vi "Create Three Input  Data Table.vi"(8 "错误输入（无错误）":errorcluster, 9 "Result":bool[](array[boolean]), 10 "Data":bool[][](array[boolean]), 11 "Data Table Ref In":refnum<vi>) -> (0 "错误输出":errorcluster, 3 "Data Table Ref Out":refnum<vi>)   [LabVIEW 2012]
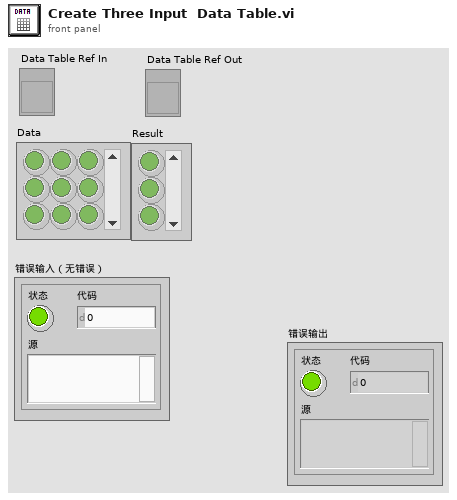
[diagram p1: front panel]
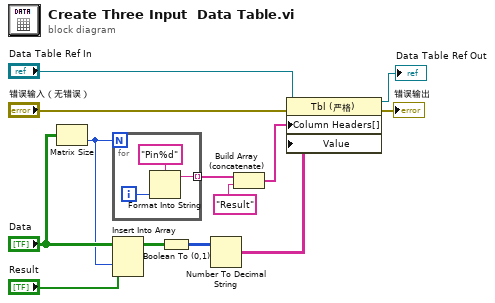
[diagram p0: block diagram]
diagram:
  n1 = Matrix Size(0:"Data") -> (2:w1:i32)  [unwired: 1 out]
  n2 = for {
    N: w1 -> [_]
    tunnel: [w14] -> w12 mode=indexing
    i -> [w16]
    n3 = Format Into String(format string="Pin%d" ("格式字符串"), w16) -> (resulting string=w14:string)  [unwired: 2 in, 1 out]
  }
  n4 = Insert Into Array(array="Data", index (col)=w1, new element="Result") -> (w2:bool[][])  [unwired: 1 in]
  n5 = Boolean To (0,1)(Boolean=w2) -> (0, 1=w10:i16[][])
  n6 = Number To Decimal String(number=w10) -> (decimal integer string=w5:string[][])  [unwired: 1 in]
  n7 = Build Array (concatenate)(w12, "Result") -> (w11:string[])
  n8 = property on="属性节点" class="Tbl (严格)"(reference="Data Table Ref In", error in="错误输入（无错误）", "Column Headers[]"=w11, "Value"=w5) -> (reference out=→"Data Table Ref Out":refnum<vi>, error out=→"错误输出":errorcluster)
